vi "Insert element.vi"(0 "connection reference":T1, 1 "NumberOfTesting":string, 5 "table":string, 7 "Results":dbl[](array[numeric]) format="%#_13g", 9 "SerialNumber":string, 11 "error in (no error)":errorcluster, 12 "TestingStatus":string) -> (4 "connection reference out":T1, 15 "error out":errorcluster)   [LabVIEW 2023, in "SQL Database.lvlib"]
uses:
  SQL Database.lvlib
  <vilib>/addons/database/Connection.llb/Conn ObjectReference.ctl
  <vilib>/addons/database/NI_Database_API.lvlib
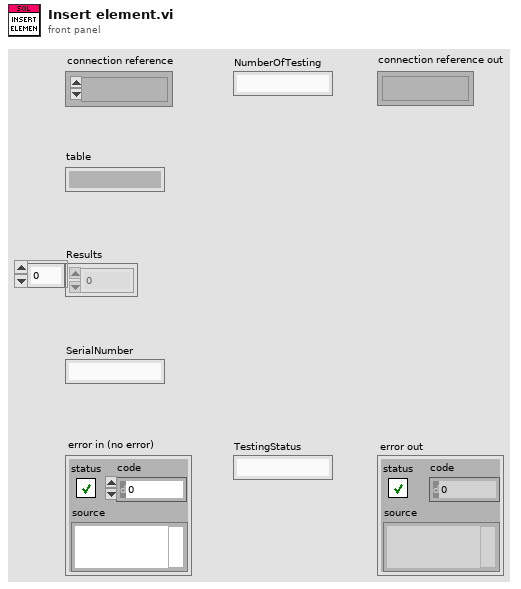
[diagram p1: front panel]
types:
  T1 = typedef "NI_Database_API.lvlib/Conn ObjectReference.ctl" = refnum<k1>
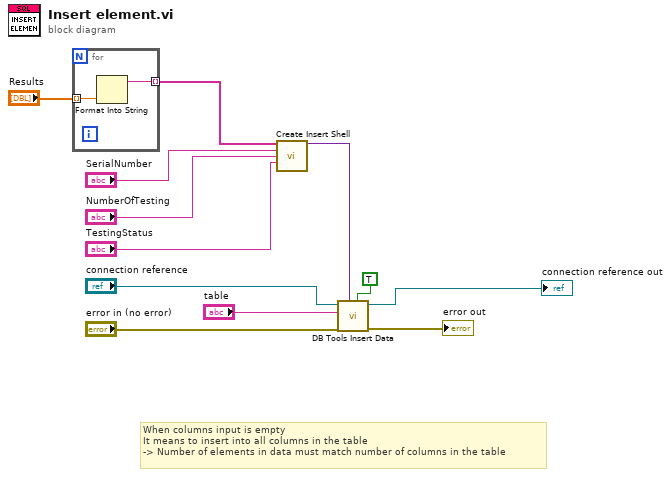
[diagram p0: block diagram]
diagram:
  # "When columns input is empty\nIt means to insert into all columns in the table\n-> Number of elements in data must match number of columns in the table"
  n1 = for {
    tunnel: "Results" -> [w14] mode=indexing
    tunnel: [w13] -> w1 mode=indexing
    n2 = Format Into String(w14) -> (resulting string=w13:string)  [unwired: 3 in, 1 out]
  }
  n3 = call "Create Insert Shell.vi"("Results"=w1, "SerialNumber"="SerialNumber", "NumberOfTesting"="NumberOfTesting", "TestingStatus"="TestingStatus") -> ("Variant"=w9:variant)  [unwired: 11 in]
  n4 = call <vilib>:"DB Tools Insert Data.vi"("create table? (F)"=TRUE, "data"=w9, "error in (no error)"="error in (no error)", "table"="table", "connection reference"="connection reference") -> ("error out"=→"error out":errorcluster, "connection reference out"=→"connection reference out":T1)  [unwired: 5 in]
